vi "PACSLI.vi"() -> ()   [LabVIEW 2017]
uses:
  <vilib>/MakerHub/LINX/Public/Peripherals/Analog/Analog Read 1 Chan.vi
  <vilib>/MakerHub/LINX/Public/Peripherals/Digital/Digital Read 1 Chan.vi
  <vilib>/MakerHub/LINX/Public/Peripherals/Digital/Digital Write 1 Chan.vi
  <vilib>/MakerHub/LINX/Public/Peripherals/Analog/Analog Read N Chans.vi
  <vilib>/MakerHub/LINX/Public/Peripherals/Digital/Digital Read N Chans.vi
  <vilib>/MakerHub/LINX/Public/Peripherals/Digital/Digital Write N Chans.vi
  <vilib>/MakerHub/LINX/Private/Local IO/LinxAnalogRead.vi
  <vilib>/MakerHub/LINX/Public/Utilities/Check Channel.vi
  <vilib>/MakerHub/LINX/Private/Local IO/LinxDigitalRead.vi
  <vilib>/MakerHub/LINX/Private/Local IO/LinxDigitalWrite.vi
  <vilib>/MakerHub/LINX/Public/Utilities/Open Serial.vi
  <vilib>/MakerHub/LINX/Private/Utilties/Generate Error.vi
  <vilib>/MakerHub/LINX/LMH-LINX.lvlib
panel:
  in  "Tab Control":enum32{"Page 1", "Page 2"}(tab)
  in  "Numeric Control 5":dbl
  in  "Numeric Control 4":dbl
  in  "Numeric Control 3":dbl
  in  "Numeric Control 2":dbl
  in  "Numeric Control":dbl
  in  "DI Channel":u8
  out "DI Value":bool
  in  "Output Value":bool
  in  "DO Channel":u8
  out "Voltage":dbl
  in  "Direction input":bool
  in  "Maximum steps":i32
  in  "Detector 1":bool
  in  "Detector 2":bool
  in  "Detector 3":bool
  in  "Detector 6":bool
  in  "Detector 4":bool
  in  "Detector 5":bool
  in  "UART Channel (0)":u8
  in  "ENA channel":u8
  in  "Photogate channel":u8
  in  "PUL channel":u8
  in  "DIR channel":u8
  in  "stop":bool
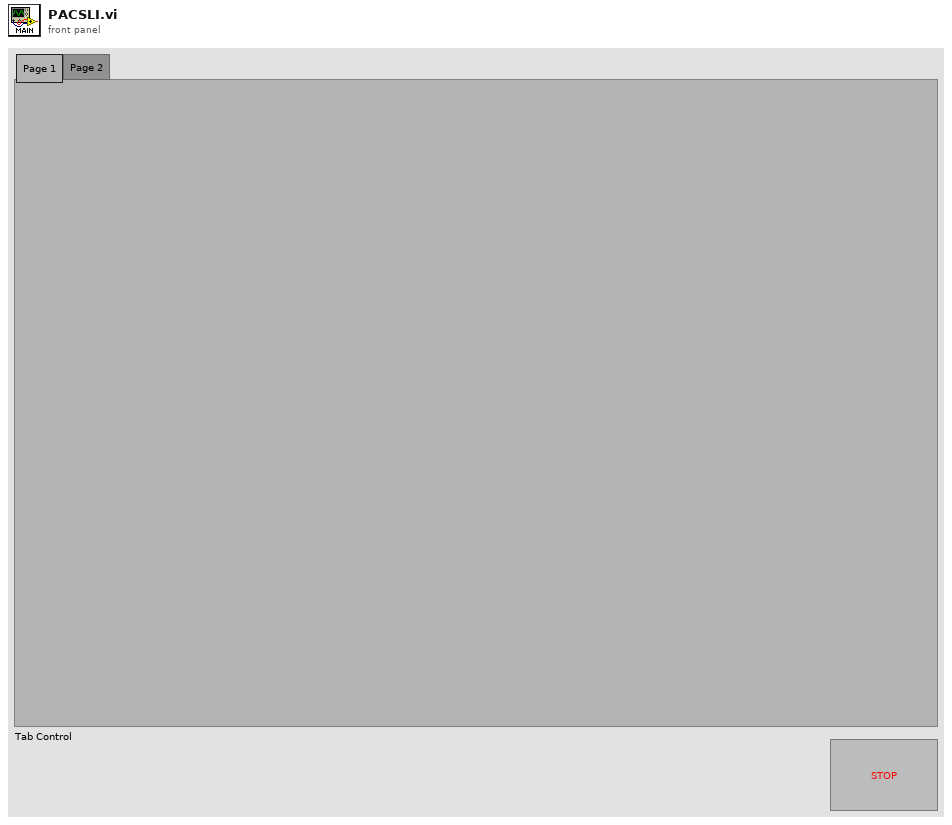
[diagram p1: front panel]
types:
  T1 = typedef "LMH-LINX.lvlib/LINX Ref.ctl" = cluster{"IO":T2, "Interface":T3, "LINX Device Config":T4}
  T2 = typedef "LMH-LINX.lvlib/Platform.ctl" = enum16{"Remote", "Local"}
  T3 = typedef "LMH-LINX.lvlib/Interface.ctl" = enum16{"Serial", "TCP"}
  T4 = typedef "LMH-LINX.lvlib/Device.lvlib/LINX Device Config.ctl" = cluster{"Interface":T3, "COM Port":refnum<visa-resource-name>, "TCP Configuration":T5, "Device Family":u8, "Device ID":u8, "Device Name":string, "TCP Ref":refnum<k5>, "Channels":T6}
  T5 = typedef "LMH-LINX.lvlib/Device.lvlib/TCP Config.ctl" = cluster{"IP Address":string, "Port":u16}
  T6 = typedef "LMH-LINX.lvlib/Channels.ctl" = cluster{"DI":u8[], "DO":u8[], "AI":u8[], "AO":u8[], "PWM":u8[], "QE":u8[], "UART":u8[], "I2C 2":u8[], "SPI":u8[], "CAN":u8[], "Servo":u8[], "AI Ref (V)":dbl, "AI Resolution (Bits)":u8, "AO Ref (V)":dbl, "AO Resolution (Bits)":u8}
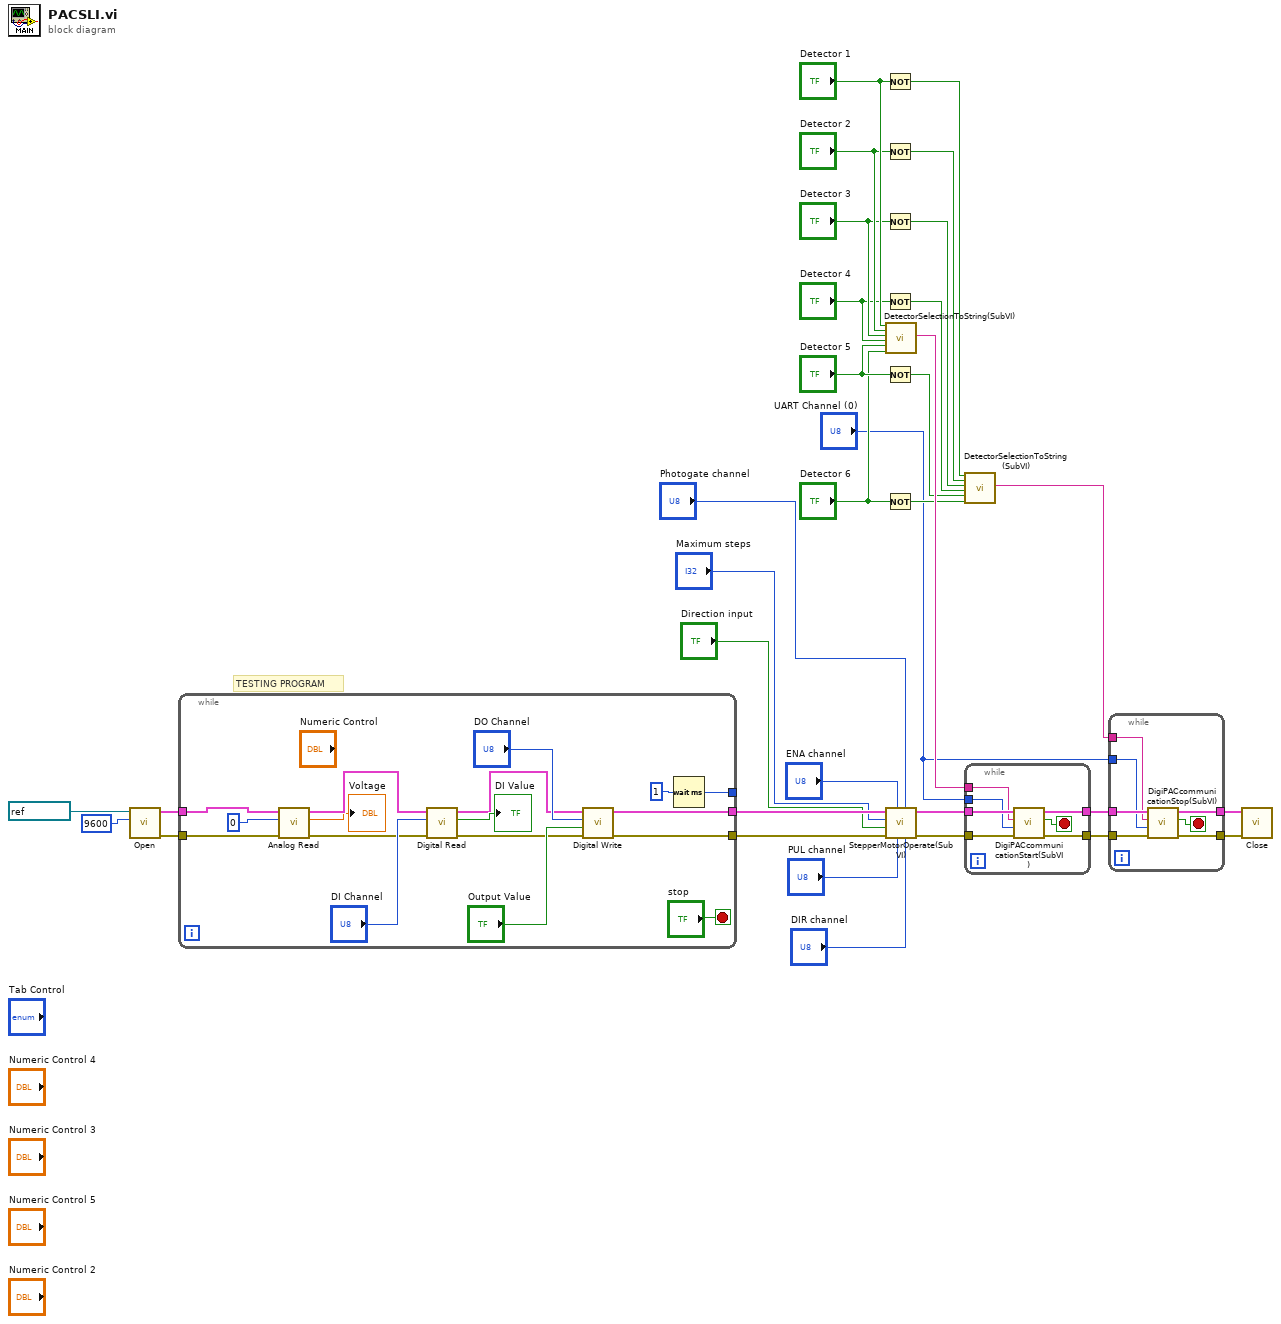
[diagram p0: block diagram]
diagram:
  # "TESTING PROGRAM"
  n1 = call-poly <vilib>:"Open.vi"("Baud Rate Override"=u32 9600, "Serial Port"=refnum<visa-resource-name> "COM3") -> ("Error Out"=w30:errorcluster, "LINX Resource"=w31:T1)  [unwired: 7 in, 1 out]
  n2 = while {
    tunnel: w31 -> [w41]
    tunnel: [w44] -> w10
    tunnel: w30 -> [w39]
    tunnel: [w42] -> w9
    tunnel: [w36] -> _
    stop <- "stop" stop-if-true
    n3 = call-poly <vilib>:"Analog Read.vi"("Error In"=w39, "Analog Channel"=u8 0, "LINX Resource"=w41) -> ("Error Out"=w38:errorcluster, "Voltage"=→"Voltage":dbl, "LINX Resource"=w40:T1)  [unwired: 5 in, 1 out]
    n4 = call-poly <vilib>:"Digital Read.vi"("Error In"=w38, "DI Channel"="DI Channel", "LINX Resource"=w40) -> ("Error Out"=w43:errorcluster, "DI Value"=→"DI Value":bool, "LINX Resource"=w45:T1)  [unwired: 6 in]
    n5 = call-poly <vilib>:"Digital Write.vi"("Error In"=w43, "Output Value"="Output Value", "DO Channel"="DO Channel", "LINX Resource"=w45) -> ("Error Out"=w42:errorcluster, "LINX Resource"=w44:T1)  [unwired: 6 in]
    n6 = Wait (ms)(milliseconds to wait=u32 1) -> (millisecond timer value=w36:u32)
  }
  n7 = Not(x="Detector 1") -> (.not. x?=w12:bool)
  n8 = Not(x="Detector 2") -> (.not. x?=w13:bool)
  n9 = Not(x="Detector 3") -> (.not. x?=w14:bool)
  n10 = Not(x="Detector 4") -> (.not. x?=w15:bool)
  n11 = Not(x="Detector 5") -> (.not. x?=w16:bool)
  n12 = Not(x="Detector 6") -> (.not. x?=w17:bool)
  n13 = call "DetectorSelectionToString(SubVI).vi"("Detector 1"="Detector 1", "Detector 2"="Detector 2", "Detector 3"="Detector 3", "Detector 4"="Detector 4", "Detector 5"="Detector 5", "Detector 6"="Detector 6") -> ("Output strting"=w29:string)  [unwired: 13 in]
  n14 = call "StepperMotorOperate(SubVI).vi"("DIR channel"="DIR channel", "Photogate channel"="Photogate channel", "PUL channel"="PUL channel", "ENA channel"="ENA channel", "error in (no error)"=w9, "Direction input"="Direction input", "Maximum steps\ninput"="Maximum steps", "LINX Resource in"=w10) -> ("error out"=w5:errorcluster, "LINX Resource out"=w6:T1)  [unwired: 2 in]
  n15 = call "DetectorSelectionToString(SubVI).vi"("Detector 1"=w12, "Detector 2"=w13, "Detector 3"=w14, "Detector 4"=w15, "Detector 5"=w16, "Detector 6"=w17) -> ("Output strting"=w24:string)  [unwired: 13 in]
  n16 = while {
    tunnel: w6 -> [w57]
    tunnel: w5 -> [w56]
    tunnel: w29 -> [w55]
    tunnel: [w54] -> w26
    tunnel: [w53] -> w25
    tunnel: "UART Channel (0)" -> [w51]
    stop <- w52 stop-if-true
    n17 = call "DigiPACcommunicationStart(SubVI).vi"("error in (no error)"=w56, "UART Channel (0)"=w51, "Detector input"=w55, "LINX Resource in"=w57) -> ("error out"=w53:errorcluster, "Measurement started?"=w52:bool, "LINX Resource out"=w54:T1)  [unwired: 5 in]
  }
  n18 = while {
    tunnel: [w63] -> w28
    tunnel: [w62] -> w27
    tunnel: w26 -> [w61]
    tunnel: w25 -> [w60]
    tunnel: w24 -> [w59]
    tunnel: "UART Channel (0)" -> [w58]
    stop <- w64 stop-if-true
    n19 = call "DigiPACcommunicationStop(SubVI).vi"("error in (no error)"=w60, "UART Channel (0)"=w58, "Detector input"=w59, "LINX Resource in"=w61) -> ("error out"=w62:errorcluster, "Measurement started?"=w64:bool, "LINX Resource out"=w63:T1)  [unwired: 5 in]
  }
  n20 = call <vilib>:"Close.vi"("Error In"=w27, "LINX Resource"=w28) -> ()  [unwired: 9 in, 1 out]
